vi "test_joystick.vi"() -> ()   [LabVIEW 2019]
panel:
  out "숫자형":i32
  out "Cluster":cluster{dbl, dbl} {"?" format="%#.1f"; "?" format="%.1f"}
  out "default val check":bool
  in  "device index":i32
  out "joystick info-out":T1
  in  "stop":bool
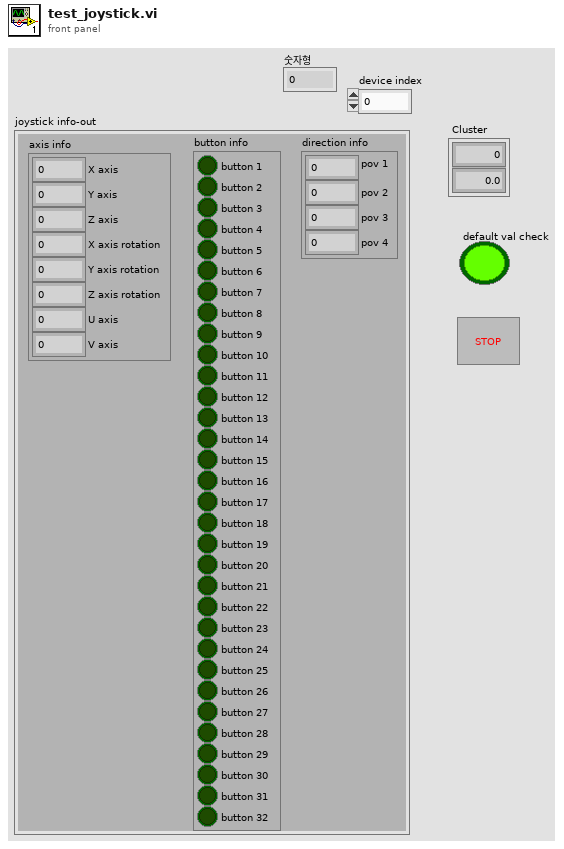
[diagram p1: front panel]
types:
  T1 = cluster{"axis info":cluster{"X axis":i32, "Y axis":i32, "Z axis":i32, "X axis rotation":i32, "Y axis rotation":i32, "Z axis rotation":i32, "U axis":i32, "V axis":i32}, "button info":cluster{"button 1":bool, "button 2":bool, "button 3":bool, "button 4":bool, "button 5":bool, "button 6":bool, "button 7":bool, "button 8":bool, "button 9":bool, "button 10":bool, "button 11":bool, "button 12":bool, "button 13":bool, "button 14":bool, "button 15":bool, "button 16":bool, "button 17":bool, "button 18":bool, "button 19":bool, "button 20":bool, "button 21":bool, "button 22":bool, "button 23":bool, "button 24":bool, "button 25":bool, "button 26":bool, "button 27":bool, "button 28":bool, "button 29":bool, "button 30":bool, "button 31":bool, "button 32":bool}, "direction info":cluster{"pov 1":i32, "pov 2":i32, "pov 3":i32, "pov 4":i32}}
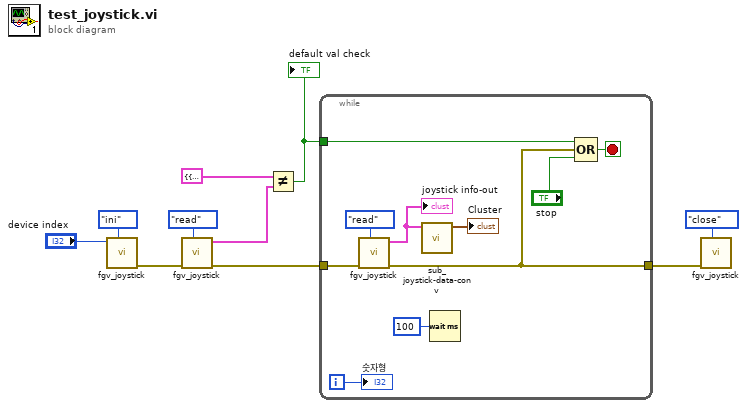
[diagram p0: block diagram]
diagram:
  n1 = call "fgv_joystick.vi"("cmd"=enum16{"ini", "read", "close"}."ini", "device index"="device index") -> ("error out"=w5:errorcluster)  [unwired: 8 in, 1 out]
  n2 = call "fgv_joystick.vi"("cmd"=enum16{"ini", "read", "close"}."read", "error in"=w5) -> ("error out"=w4:errorcluster, "joystick info-out"=w2:T1)  [unwired: 8 in]
  n3 = Not Equal?(x=T1 {"axis info"={"X axis"=0, "Y axis"=-256, "Z axis"=0, "X axis rotation"=0, "Y axis rotation"=0, "Z axis rotation"=-256, "U axis"=0, "V axis"=0}, "button info"={"button 1"=FALSE, "button 2"=FALSE, "button 3"=FALSE, "button 4"=FALSE, "button 5"=FALSE, "button 6"=FALSE, "button 7"=FALSE, "button 8"=FALSE, "button 9"=FALSE, "button 10"=FALSE, "button 11"=FALSE, "button 12"=FALSE, "button 13"=FALSE, "button 14"=FALSE, "button 15"=FALSE, "button 16"=FALSE, "button 17"=FALSE, "button 18"=FALSE, "button 19"=FALSE, "button 20"=FALSE, "button 21"=FALSE, "button 22"=FALSE, "button 23"=FALSE, "button 24"=FALSE, "button 25"=FALSE, "button 26"=FALSE, "button 27"=FALSE, "button 28"=FALSE, "button 29"=FALSE, "button 30"=FALSE, "button 31"=FALSE, "button 32"=FALSE}, "direction info"={"pov 1"=-1, "pov 2"=-1, "pov 3"=-1, "pov 4"=-1}} ("joystick info-out 2"), y=w2) -> (x != y?=w1:bool)
  "default val check" <- w1
  n4 = while {
    tunnel: [w17] -> w8
    tunnel: w4 -> [w18]
    tunnel: w1 -> [w16]
    i -> [w11]
    stop <- w14 stop-if-true
    n5 = call "fgv_joystick.vi"("cmd"=enum16{"ini", "read", "close"}."read", "error in"=w18) -> ("error out"=w17:errorcluster, "joystick info-out"=w13:T1)  [unwired: 8 in]
    "joystick info-out" <- w13
    n6 = call "sub_joystick-data-conv.vi"("joystick info-in"=w13) -> ("opval"=→"Cluster":cluster{dbl, dbl})  [unwired: 10 in]
    n7 = Wait (ms)(milliseconds to wait=u32 100) -> ()  [unwired: 1 out]
    n8 = Compound Arithmetic op=OR(w16, w17, "stop") -> (w14:bool)
    "숫자형" <- w11
  }
  n9 = call "fgv_joystick.vi"("cmd"=enum16{"ini", "read", "close"}."close", "error in"=w8) -> ()  [unwired: 8 in, 2 out]
